vi "Control Test Bench.vi"() -> ()   [LabVIEW 2020]
uses:
  Title - Type Def.ctl
  Employee Record - Strict Type Def.ctl
  Employee Record - Type Def.ctl
panel:
  in  "Employee Record - Type Def 2":T1={"Title"=enum."Mr", "First Name"="Jennifer", "Preferred Name"="Jenny", "Surname"="Swift", "Department"=enum."Finance", "Employment Status"=enum."Part Time", "Start Date"=timestamp(3565024425.501588 s since 1904-01-01), "Normal Working Location"=enum."Working in Office"} {"Start Date" format="%<%x %.3X>T"}
  in  "Employee Record -  Strict Type Def 2":T3={"Title"=enum."Mr", "First Name"="Jennifer", "Preferred Name"="Jenny", "Surname"="Swift", "Department"=enum."Finance", "Employment Status"=enum."Part Time", "Start Date"=timestamp(3565024425.501588 s since 1904-01-01), "Normal Working Location"=enum."Working in Office"} {"Start Date" format="%<%x %.3X>T"}
  in  "Employee Record - Control 2":T4={"Title"=enum."Mr", "First Name"="Jennifer", "Preferred Name"="Jenny", "Surname"="Swift", "Department"=enum."Finance", "Employment Status"=enum."Part Time", "Start Date"=timestamp(3565024425.501588 s since 1904-01-01), "Normal Working Location"=enum."Working in Office"} {"Start Date" format="%<%x %.3X>T"}
  in  "Employee Record - Type Def":T1={"Title"=enum."Mr", "First Name"="Jennifer", "Preferred Name"="Jenny", "Surname"="Swift", "Department"=enum."Finance", "Employment Status"=enum."Part Time", "Start Date"=timestamp(3565024425.501588 s since 1904-01-01), "Normal Working Location"=enum."Working in Office"} {"Start Date" format="%<%x %.3X>T"}
  in  "Employee Record -  Strict Type Def":T3={"Title"=enum."Mr", "First Name"="Jennifer", "Preferred Name"="Jenny", "Surname"="Swift", "Department"=enum."Finance", "Employment Status"=enum."Part Time", "Start Date"=timestamp(3565024425.501588 s since 1904-01-01), "Normal Working Location"=enum."Working in Office"} {"Start Date" format="%<%x %.3X>T"}
  in  "Employee Record - Control":T5={"Title"=enum."Mr", "First Name"="Jennifer", "Last Name"="Swift", "Department"=enum."Finance", "Employment Status"=enum."Part Time", "Start Date"=timestamp(3565024425.501588 s since 1904-01-01), "Normal Working Location"=enum."Working in Office"} {"Start Date" format="%<%x %.3X>T"}
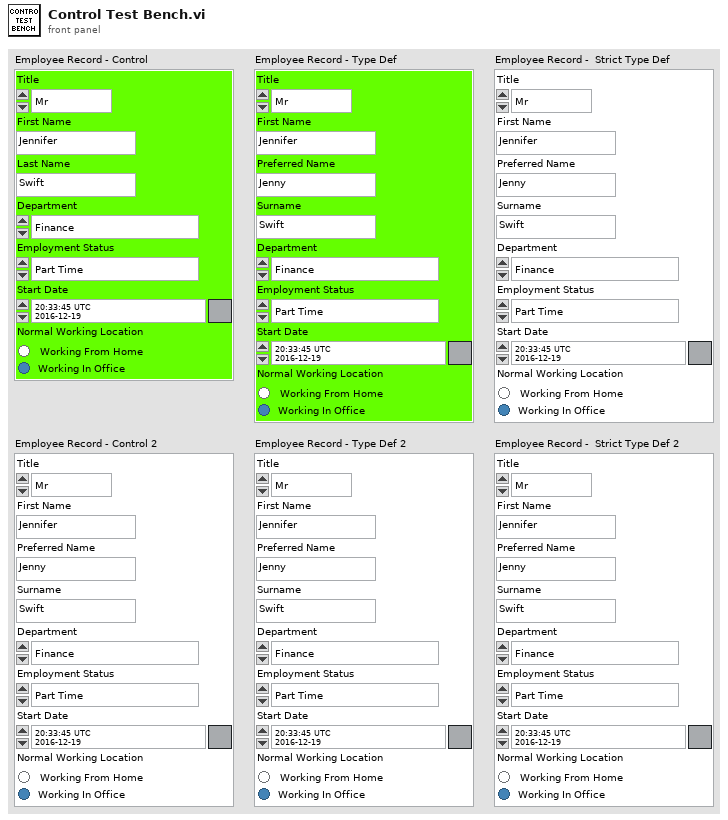
[diagram p1: front panel]
types:
  T1 = typedef "Employee Record - Type Def.ctl" = cluster{"Title":T2, "First Name":string, "Preferred Name":string, "Surname":string, "Department":enum16{"Research and Development", "Technical Support", "Sales", "Management", "Finance", "Other"}, "Employment Status":enum16{"Full Time", "Part Time", "No Longer Employed", "Probation", "Other"}, "Start Date":timestamp, "Normal Working Location":enum32{"Working From Home", "Working in Office"}}
  T2 = typedef "Title - Type Def.ctl" = enum16{"Mr", "Mrs", "Ms", "Mx", "Miss", "Sir", "Dame", "Other"}
  T3 = typedef "Employee Record - Strict Type Def.ctl" = cluster{"Title":T2, "First Name":string, "Preferred Name":string, "Surname":string, "Department":enum16{"Research and Development", "Technical Support", "Sales", "Management", "Finance", "Other"}, "Employment Status":enum16{"Full Time", "Part Time", "No Longer Employed", "Probation", "Other"}, "Start Date":timestamp, "Normal Working Location":enum32{"Working From Home", "Working in Office"}}
  T4 = cluster{"Title":T2, "First Name":string, "Preferred Name":string, "Surname":string, "Department":enum16{"Research and Development", "Technical Support", "Sales", "Management", "Finance", "Other"}, "Employment Status":enum16{"Full Time", "Part Time", "No Longer Employed", "Probation", "Other"}, "Start Date":timestamp, "Normal Working Location":enum32{"Working From Home", "Working in Office"}}
  T5 = cluster{"Title":T2, "First Name":string, "Last Name":string, "Department":enum16{"Research and Development", "Technical Support", "Sales", "Management", "Finance", "Other"}, "Employment Status":enum16{"Full Time", "Part Time", "No Longer Employed", "Probation", "Other"}, "Start Date":timestamp, "Normal Working Location":enum32{"Working From Home", "Working in Office"}}
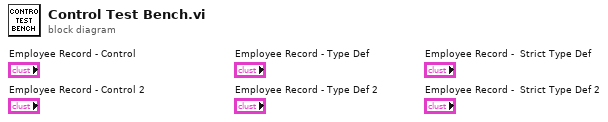
[diagram p0: block diagram]
diagram:
